vi "test2.vi"() -> ()   [LabVIEW 2016]
uses:
  <vilib>/Instr/_visa.llb/VISA Configure Serial Port (Instr).vi
panel:
  in  "stop":bool
  out "concatenated string":string
  out "hex integer string":string
  in  "Установка значения дв":bool
  out "Boolean":bool
  in  "Минуты":u64 max=16777215
  in  "DTR Write":bool
  in  "RTS Write":bool
  in  "VISA resource name":refnum<visa-resource-name>
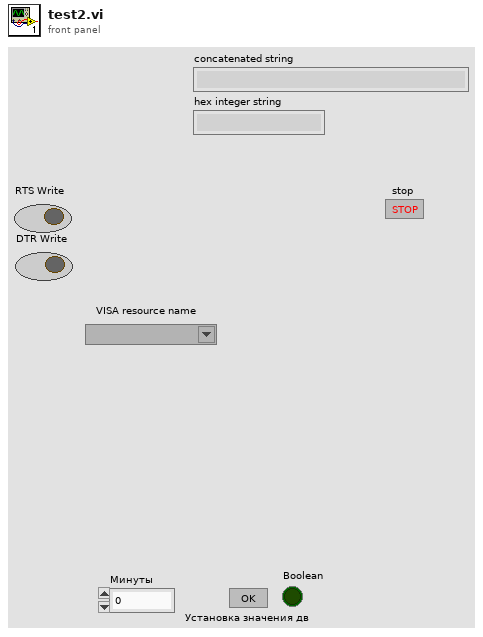
[diagram p1: front panel]
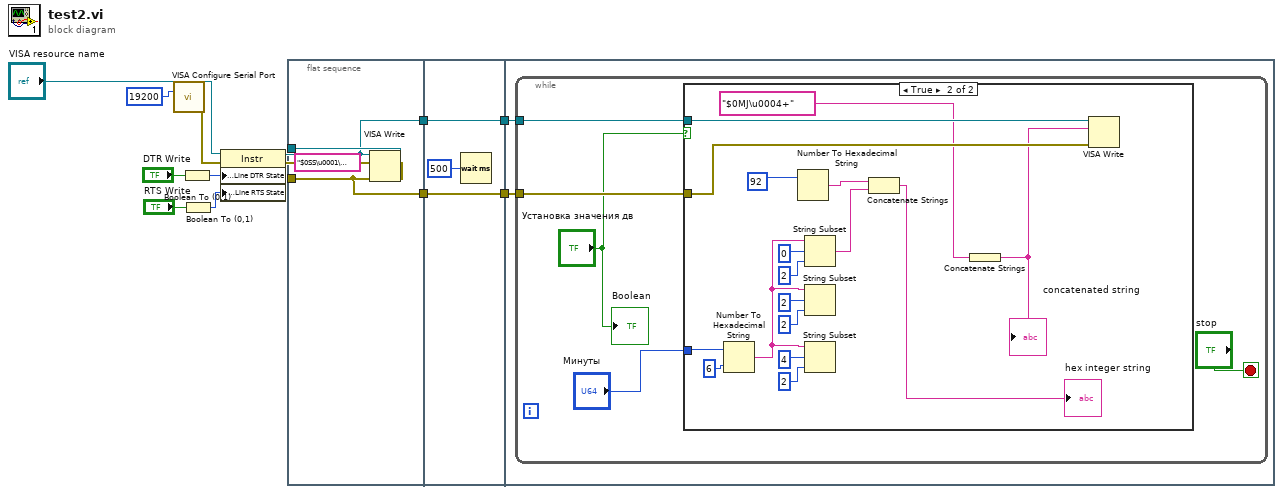
[diagram p0: block diagram]
diagram:
  n1 = call-poly "VISA Configure Serial Port"("VISA resource name"="VISA resource name", "baud rate (9600)"=u32 19200) -> ("VISA resource name out"=w4:refnum<visa-resource-name>, "error out"=w3:errorcluster)  [unwired: 12 in]
  n2 = Boolean To (0,1)(Boolean="DTR Write") -> (0, 1=w5:i16)
  n3 = Boolean To (0,1)(Boolean="RTS Write") -> (0, 1=w7:i16)
  n4 = property class="Instr"(reference=w4, error in=w3, "Serial Settings:Modem Line Settings:Line DTR State"=w5, "Serial Settings:Modem Line Settings:Line RTS State"=w7) -> (reference out=w2:refnum<visa-resource-name>, error out=w1:errorcluster)
  n5 = flat-sequence {
    tunnel: w2 -> [w16]
    tunnel: w1 -> [w15]
    tunnel: [w16] -> w14
    tunnel: [w15] -> w13
    tunnel: [w19] -> w12
    tunnel: w14 -> [w19]
    tunnel: w13 -> [w18]
    tunnel: [w18] -> w11
    tunnel: w12 -> [w22]
    tunnel: w11 -> [w21]
    frame #0 {
      n6 = VISA Write(VISA resource name=w16, write buffer="$0SS\u0001\u0010", error in (no error)=w15) -> ()  [unwired: 3 out]
    }
    frame #1 {
      n7 = Wait (ms)(milliseconds to wait=u32 500) -> ()  [unwired: 1 out]
    }
    frame #2 {
      n8 = while {
        tunnel: w22 -> [w26]
        tunnel: w21 -> [w25]
        stop <- "stop" stop-if-true
        n9 = case shown="True" "Установка значения дв" {
          tunnel: w26 -> [_ w44]
          tunnel: w25 -> [_ w43]
          tunnel: "Минуты" -> [_ w41]
          frame False {
          }
          frame True {
            n10 = Number To Hexadecimal String(1:i16 6 ("width (-)"), 2:w41) -> (0:w34:string)
            n11 = Number To Hexadecimal String(2:92) -> (0:w30:string)  [unwired: 1 in]
            n12 = String Subset(string=w34, offset (0)=i16 0 ("width (-)"), length (rest)=i16 2 ("width (-)")) -> (substring=w31:string)
            n13 = String Subset(string=w34, offset (0)=i16 2 ("width (-)"), length (rest)=i16 2 ("width (-)")) -> ()  [unwired: 1 out]
            n14 = String Subset(string=w34, offset (0)=i16 4 ("width (-)"), length (rest)=i16 2 ("width (-)")) -> ()  [unwired: 1 out]
            n15 = Concatenate Strings(w30, w31) -> (→"hex integer string":string)
            n16 = Concatenate Strings("$0MJ\u0004+" ("write buffer")) -> (w33:string)
            "concatenated string" <- w33
            n17 = VISA Write(VISA resource name=w44, write buffer=w33, error in (no error)=w43) -> ()  [unwired: 3 out]
          }
        }
        "Boolean" <- "Установка значения дв"
      }
    }
  }
